vi "Place Control on VI.vi"(0 "VI in":refnum<vi>, 7 "Control in":refnum<vi>, 11 "error in (no error)":errorcluster) -> (4 "VI out":refnum<vi>, 8 "Control out":refnum<vi>, 15 "error out":errorcluster)   [LabVIEW 2017, in "Variant Control Scripting.lvlib"]
uses:
  Variant Control Scripting/Source/Variant Control Scripting.lvlib
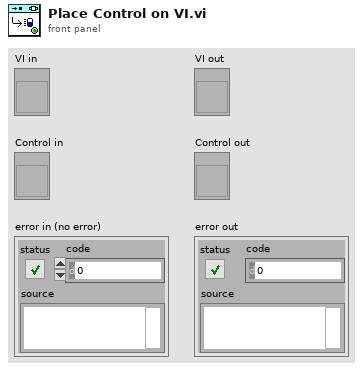
[diagram p1: front panel]
types:
  T1 = enum8{"Probe", "Diagram", "Panel Control", "3D Panel Control", "Dialog Panel Control", "Panel Indicator", "3D Panel Indicator", "Dialog Panel Indicator", "Power PC Control", "Power PC Indicator", "Silver Control", "Silver Indicator"}
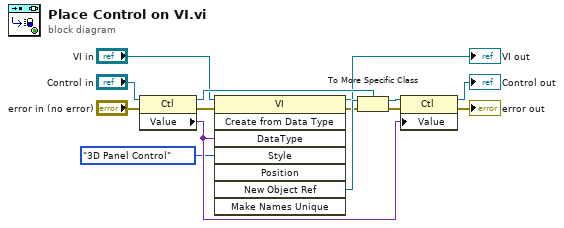
[diagram p0: block diagram]
diagram:
  n1 = property class="Ctl"(reference="Control in", error in="error in (no error)") -> (reference out=w13:refnum<vi>, error out=w8:errorcluster, "Value"=w14:variant)
  n2 = invoke class="VI" method="Create from Data Type"(reference="VI in", error in=w8, "DataType"=w14, "Style"=T1."3D Panel Control") -> (reference out=→"VI out":refnum<vi>, error out=w7:errorcluster, "New Object Ref"=w11:refnum<vi>)  [unwired: 4 in, 5 out]
  n3 = To More Specific Class(target class=w13, reference=w11, error in=w7) -> (specific class reference=w12:refnum<vi>, error out=w6:errorcluster)
  n4 = property class="Ctl"(reference=w12, error in=w6, "Value"=w14) -> (reference out=→"Control out":refnum<vi>, error out=→"error out":errorcluster)
